vi "Cycle End.vi"(8 "error in (no error)":errorcluster, 11 "Framework in":refnum<class "Framework.lvclass">) -> (0 "error out":errorcluster, 3 "Framework out":refnum<class "Framework.lvclass">)   [LabVIEW 2019, in "DSF Core.lvlib" / "Framework.lvclass"]
uses:
  Framework.lvclass
  Framework.lvclass/Framework.ctl
  Plugin/Plugin.lvclass/Plugin.ctl
  Timing/Timing.lvclass/Timing.ctl
  Performance/Performance.lvclass/Performance.ctl
  <vilib>/NI/Memory Manager/Classes/Pointer/Pointer.lvclass/Pointer.ctl
  Framework Status/Framework Status.lvclass/Framework Status.ctl
  Performance/Write Timing Status.vi
  Status/Write Status.vi
  Performance/Get Timing Status.vi
  Framework Status/Get Framework Pointer.vi
  Plugin/Increment Iteration.vi
  Timing Status/Write Timing Status.vi
  <vilib>/NI/Memory Manager/Classes/Pointer/Get Address.vi
  Status/Status Size.vi
  <vilib>/NI/Memory Manager/Classes/Pointer/Check Null Pointer.vi
  <vilib>/NI/Memory Manager/Classes/Pointer/Check Size.vi
  Timing/Get Iteration.vi
  Status/Subset Status.vi
  Timing/Increment Iteration.vi
  Timing Status/Timing Status Size.vi
  <vilib>/NI/Memory Manager/Classes/Pointer/Errors.vi
  <vilib>/NI/Memory Manager/Classes/Pointer/Null Pointer.vi
  <vilib>/NI/Memory Manager/Classes/Pointer/Is Null.vi
  <vilib>/NI/Memory Manager/Classes/Pointer/Out of Bounds.vi
  <vilib>/NI/Memory Manager/Classes/Pointer/Get Size.vi
  <vilib>/NI/Memory Manager/Classes/Pointer/Subset.vi
  <vilib>/NI/Memory Manager/Classes/Pointer/Create Error.vi
  <vilib>/NI/Memory Manager/VIs/Write String to Source.vi
  <vilib>/NI/Memory Manager/Classes/Pointer/Write Pointer Size to Error.vi
  <vilib>/NI/Memory Manager/VIs/Write Numeric to Source.vi
  <vilib>/NI/Memory Manager/VIs/Write Numeric Scalar to Source (Base10 U64).vi
  <vilib>/NI/Memory Manager/Classes/Pointer/Encapsulate.vi
  <vilib>/NI/Memory Manager/Classes/Pointer/Check Length.vi
  <vilib>/NI/Memory Manager/VIs/New Error Cluster.vi
  <vilib>/NI/Memory Manager/VIs/New Error Cluster (512B).vi
  <vilib>/NI/Memory Manager/VIs/Set Error Status.vi
  <vilib>/NI/Memory Manager/VIs/Set Error Code.vi
  <vilib>/NI/Memory Manager/VIs/Set Error Source.vi
  <vilib>/NI/Memory Manager/Constants/Constants.vi
  <vilib>/NI/Memory Manager/Constants/Library Name.vi
  <vilib>/NI/Memory Manager/Classes/Pointer/Pointer Error Info.vi
  <vilib>/NI/Memory Manager/Constants/Pointer Class Name.vi
  <vilib>/NI/Memory Manager/Classes/Pointer/Set Size.vi
  <vilib>/NI/Memory Manager/Classes/Pointer/Set Address.vi
  <vilib>/NI/Memory Manager/Classes/Pointer/Set Internal.vi
  <vilib>/NI/Memory Manager/Classes/Pointer/Check Bounds (Pointer).vi
  Timing Status/Timing Status Pointer.lvclass
  C:/Program Files (x86)/National Instruments/LabVIEW 2019/vi.lib/NI/Memory Manager/Classes/Pointer/Pointer.lvclass
  Status/Status Pointer.lvclass
  Performance/Performance.lvclass
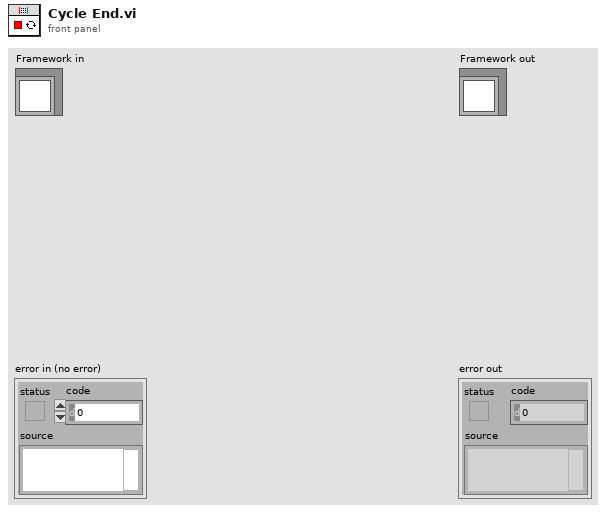
[diagram p1: front panel]
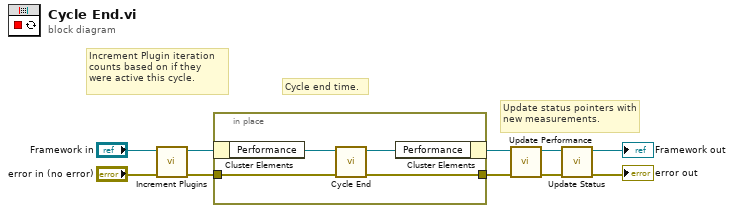
[diagram p0: block diagram]
diagram:
  # "Update status pointers with new measurements."
  # "Cycle end time."
  # "Increment Plugin iteration counts based on if they were active this cycle."
  n1 = call "Increment Plugins.vi"("error in (no error)"="error in (no error)", "Framework in"="Framework in") -> ("error out"=w1:errorcluster, "Framework out"=w2:refnum<class "Framework.lvclass">)  [unwired: 8 in]
  n2 = in-place {
    in-place-border: w1 -> [w12]
    in-place-border: [w11] -> w7
    n3 = in-place-cluster #1(w2) -> ("Performance"=w14:refnum<class "Performance.lvclass">)
    n4 = call "Cycle End.vi"("error in (no error)"=w12, "Performance in"=w14) -> ("error out"=w11:errorcluster, "Performance out"=w13:refnum<class "Performance.lvclass">)  [unwired: 8 in]
    n5 = in-place-cluster #1("Performance"=w13) -> (w8:refnum<class "Framework.lvclass">)
  }
  n6 = call "Update Performance.vi"("error in (no error)"=w7, "Framework in"=w8) -> ("error out"=w9:errorcluster, "Framework out"=w10:refnum<class "Framework.lvclass">)  [unwired: 8 in]
  n7 = call "Update Status.vi"("error in (no error)"=w9, "Framework in"=w10) -> ("error out"=→"error out":errorcluster, "Framework out"=→"Framework out":refnum<class "Framework.lvclass">)  [unwired: 8 in]
